vi "Main.vi"() -> ()   [LabVIEW 2013]
uses:
  <vilib>/Instr/_visa.llb/VISA Flush IO Buffer Mask.ctl
  <vilib>/Instr/_visa.llb/VISA Configure Serial Port (Instr).vi
panel:
  out "Roll Array":dbl[](array[numeric])
  out "Pitch Array":dbl[](array[numeric])
  out "Time for Orientation":dbl[](array[numeric])
  out "Time for Temp":dbl[](array[numeric])
  out "Heater Temp":dbl[](array[numeric])
  out "Temp 2":dbl[](array[numeric])
  out "Temp 1":dbl[](array[numeric])
  out "Start time (minutes)":dbl
  out "error out":errorcluster
  in  "error in (no error)":errorcluster
  in  "Tab Control":T1(tab)
  out "Command Recieved":bool
  in  "Reset Relays":bool
  in  "Reset Radio Check":bool
  out "Check Successful!":bool
  in  "Radio Check":bool
  out "Relay 8 Status":bool
  out "Relay 7 Status":bool
  out "Relay 6 Status":bool
  out "Relay 5 Status":bool
  out "Relay 4 Status":bool
  out "Relay 3 Status":bool
  out "Relay 2 Status":bool
  out "Relay 1 Status":bool
  in  "Relay 8":bool
  in  "Relay 7":bool
  in  "Relay 6":bool
  in  "Relay 5":bool
  in  "Relay 4":bool
  in  "Relay 3":bool
  in  "Relay 2":bool
  in  "Relay 1":bool
  out "Manual Heat Control?":bool
  out "Current Time":timestamp format="%<%I:%M:%S %p>T"
  in  "Command":u16(ring) items=["CUTDOWN"=0, "CHANGE_TRANSMIT_RATE"=1, "TURN_HEATER_ON"=2, "TURN_HEATER_OFF"=3, "MANUAL_HEATER_CONTROL"=4, "SWITCH_RELAYS"=100]
  in  "Value":u16
  out "Sensor Specifications Exceeded":bool caption="Warning"
  in  "Stop":bool
  in  "Last Recieved Packet":string
  out "Radio Connection Lost":bool caption="Alarm"
  out "Turbulence":bool caption="Warning"
  in  "Baud Rate":i32=115200
  out "Data Logging OFF":bool caption="Warning"
  in  "Packet Logging File":path
  in  "Log Recieved Packets?":bool=TRUE
  out "Time of Last Recieved Packet":timestamp format="%<%I:%M:%S %p>T"
  out "Heater On?":bool
  out "Yaw":dbl
  out "Roll":dbl
  out "Pitch":dbl
  in  "COM Port":refnum<visa-resource-name>
  in  "Send Command":bool
  in  "Interior Temperature 2":dbl(knob) scale=-60.0..40.0
  out "Relative Humidity":dbl(knob) scale=0.0..100.0
  out "Atmospheric Pressure":dbl(knob) scale=0.0..15.0
  out "Flight Duration":timestamp format="%<%H:%M:%S>T"
  out "Low Interior Temperature":bool caption="Warning"
  out "Critically Low Interior Temperature":bool caption="Alarm"
  in  "Interior Temperature 1":dbl(knob) scale=-60.0..40.0
  in  "Exterior Temperature":dbl(knob) scale=-60.0..40.0
  in  "Heater Temperature":dbl(knob) scale=-60.0..40.0
  out "Yaw":cluster{"X":dbl, "Y":dbl}[](graph)
  out "Atmospheric Pressure":cluster{"X":dbl, "Y":dbl}[](graph)
  out "Exterior Temperature":cluster{"X":dbl, "Y":dbl}[](graph)
  out "Relative Humidity":cluster{"X":dbl, "Y":dbl}[](graph)
  out "Interior Temperature":cluster{dbl[], dbl[]}[](graph)
  out "Pitch/Roll":cluster{dbl[], dbl[]}[](graph)
  in  "Save Packets":bool
  in  "Packet File":path
  out "Packets Recieved":string
  # "Current Instrument Readings"
  # "Relay Status"
  # "Control"
  # "Notes: \n + Relay 1: Tracer 1\n + Relay 2: Unused\n + Relay 3: Unused\n + Relay 4: Heater relay (control blocked)\n\n + Relays 5-8 are not currently wired"
  # "Relays"
  # "See \"Relay Status\"\n panel for relay \nassignments"
  # "Warnings and Alarms"
  # "Communication"
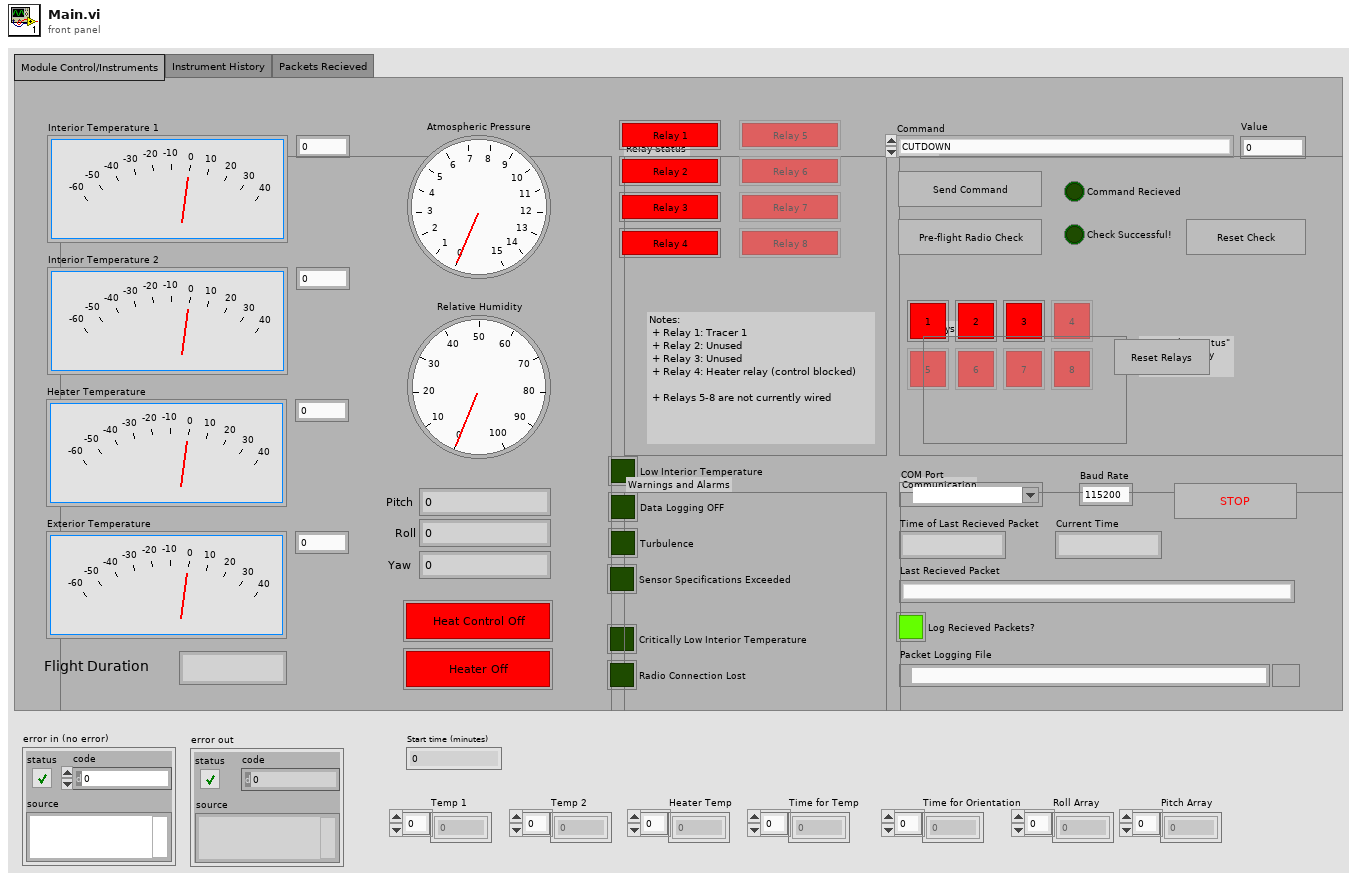
[diagram p1: front panel]
types:
  T1 = enum32{"Module Control/Instruments", "Instrument History", "Packets Recieved"}
  T2 = typedef "VISA Flush IO Buffer Mask.ctl" = u16
  T3 = enum16{"open", "replace", "create", "open or create", "replace or create", "replace or create with confirmation"}
  T4 = cluster{"Digital Interior Temperature":dbl, "Analog Interior Temperature":dbl, "Heater Temperature":dbl, "Exterior Temperature":dbl, "Humidity":dbl, "Pressure":dbl, "Pitch":dbl, "Roll":dbl, "Yaw":dbl, "Heater On?":bool, "Data Logging?":bool, "Manual Heat Control?":bool, "Turbulence":bool, "Relay 1":bool, "Relay 2":bool, "Relay 3":bool, "Relay 4":bool, "Relay 5":bool, "Relay 6":bool, "Relay 7":bool, "Relay 8":bool}
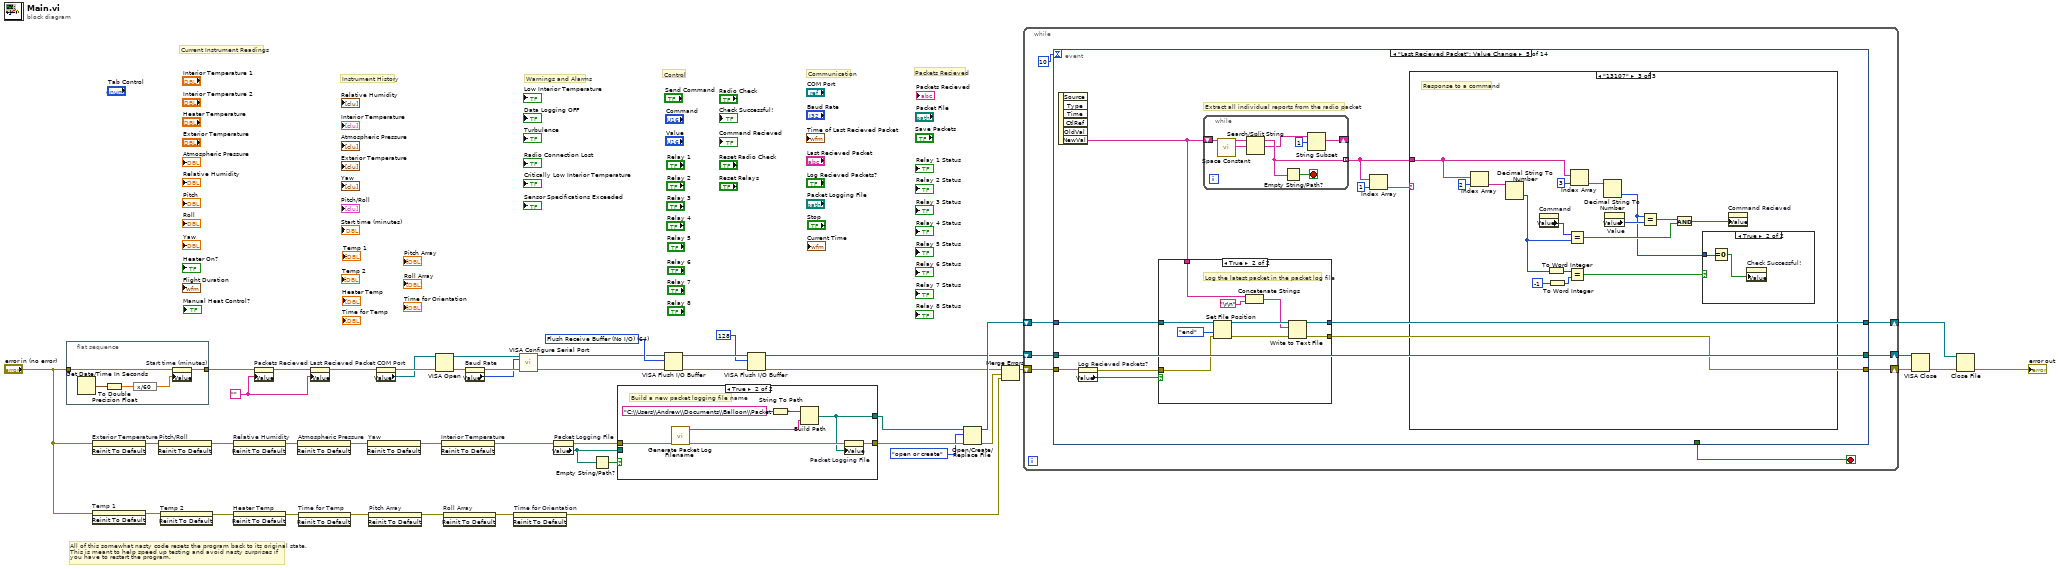
[diagram p0: block diagram]
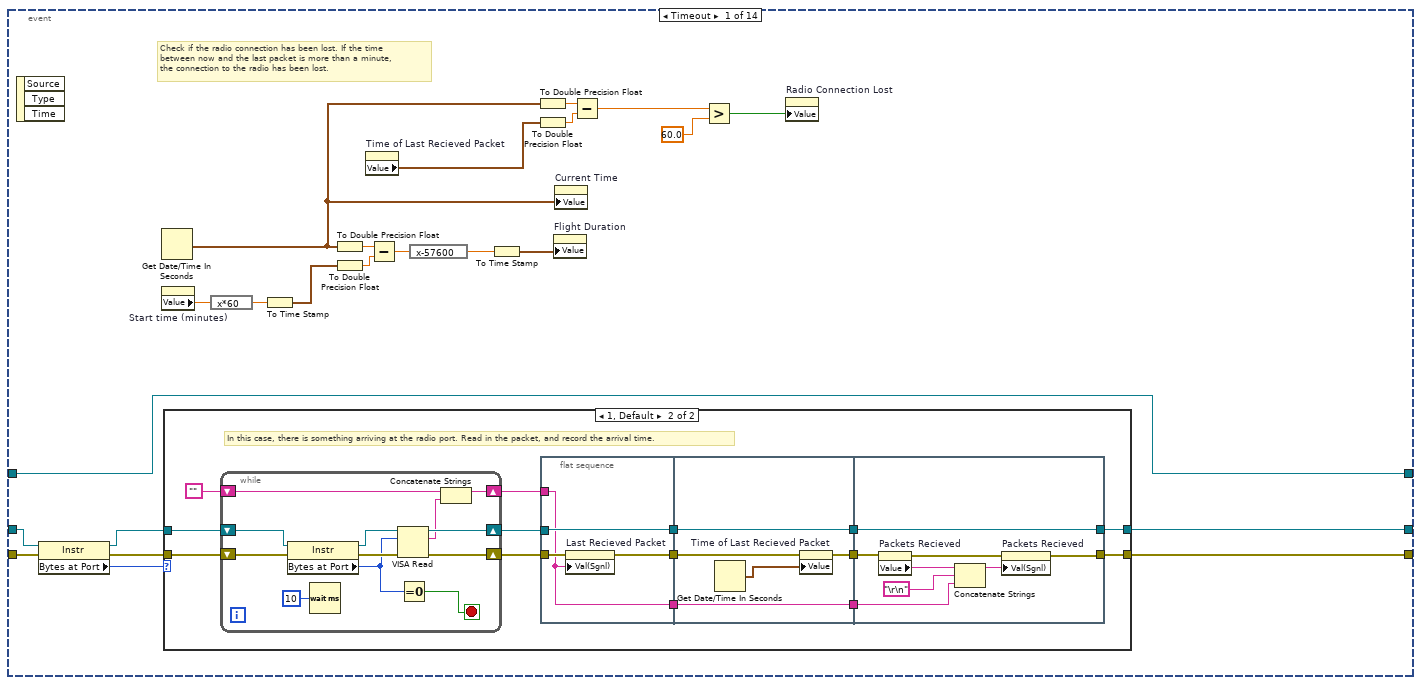
[diagram p3: hidden frame]
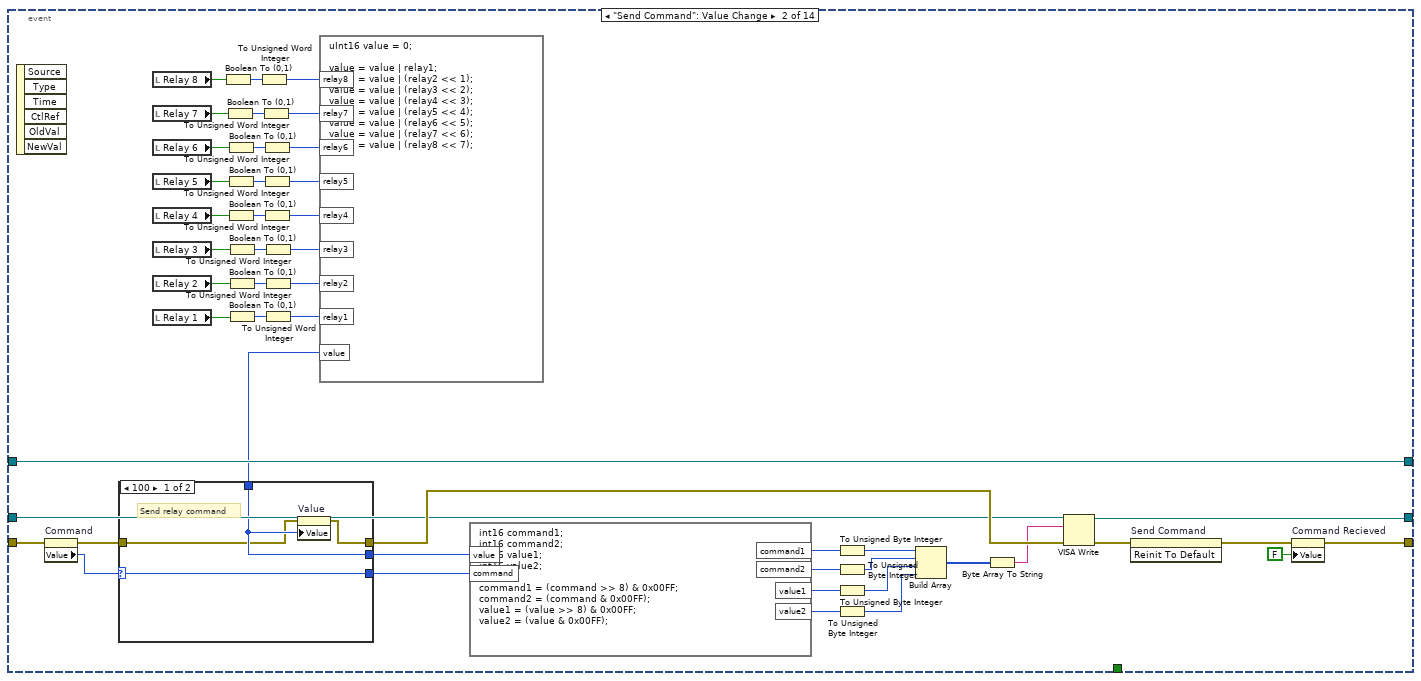
[diagram p5: hidden frame]
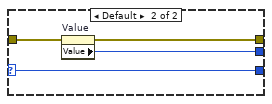
[diagram p6: hidden frame]
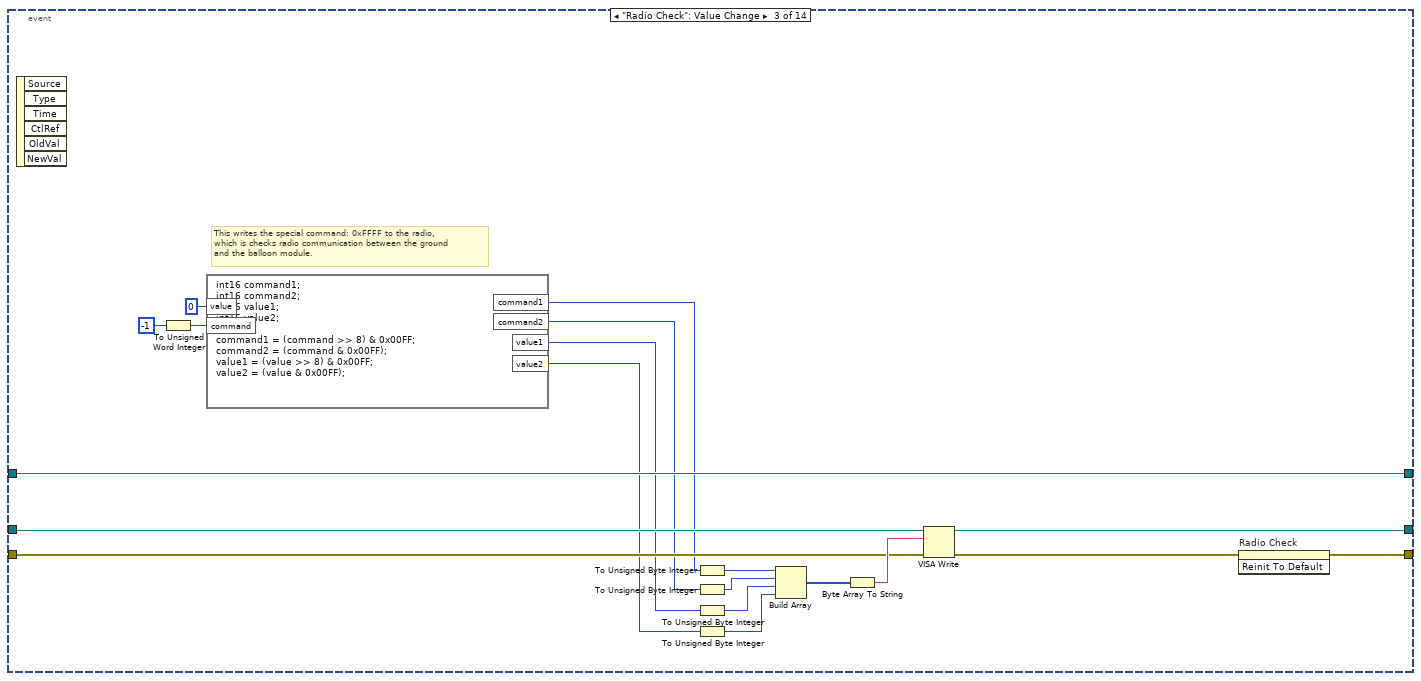
[diagram p7: hidden frame]
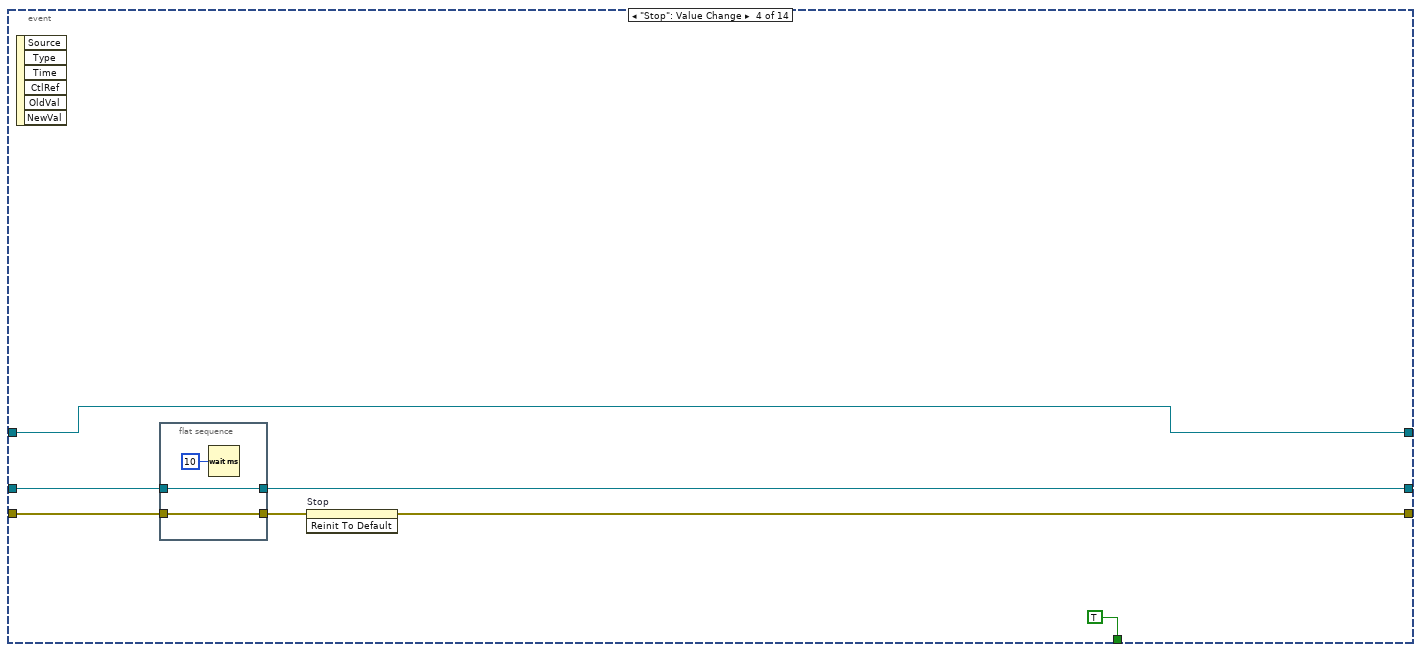
[diagram p8: hidden frame]
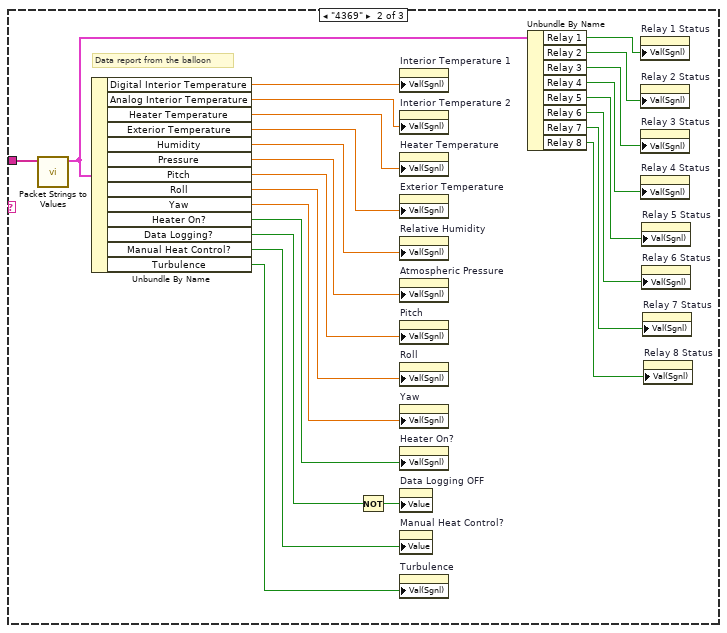
[diagram p10: hidden frame]
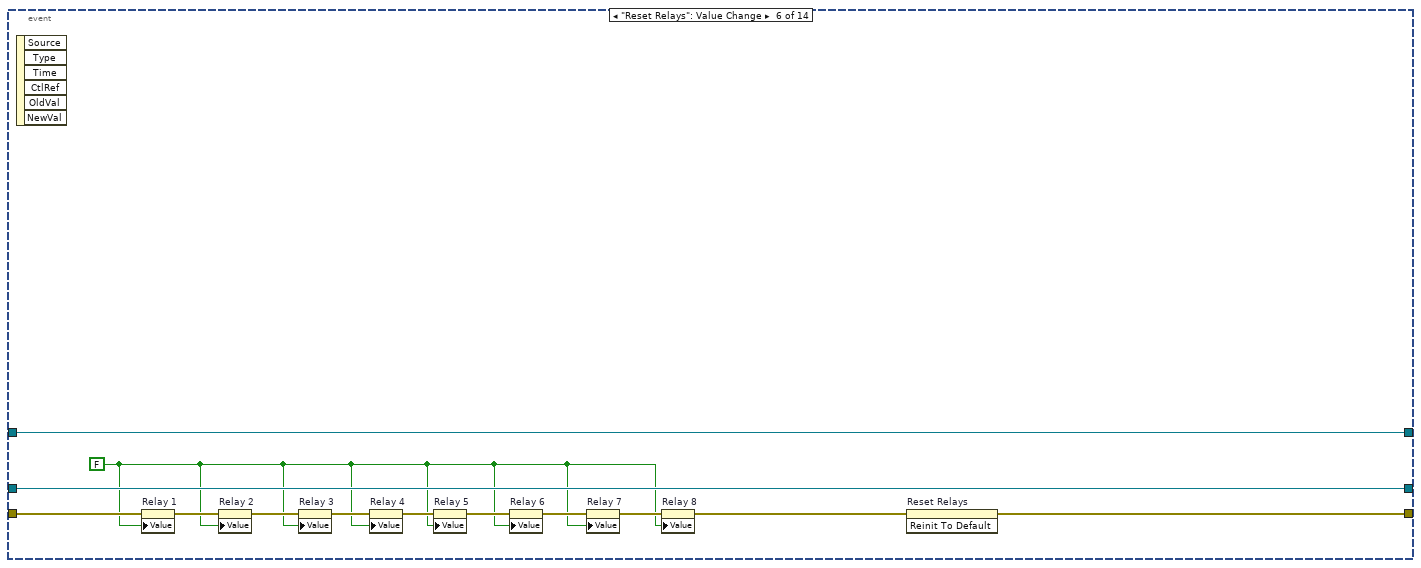
[diagram p13: hidden frame]
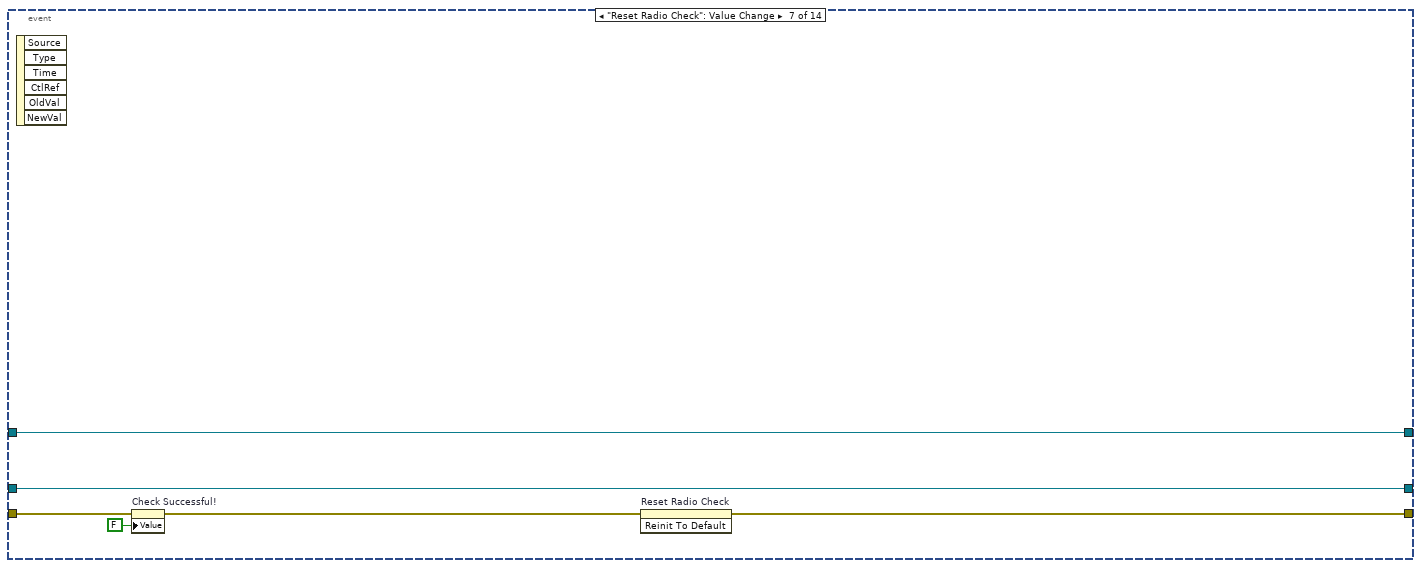
[diagram p14: hidden frame]
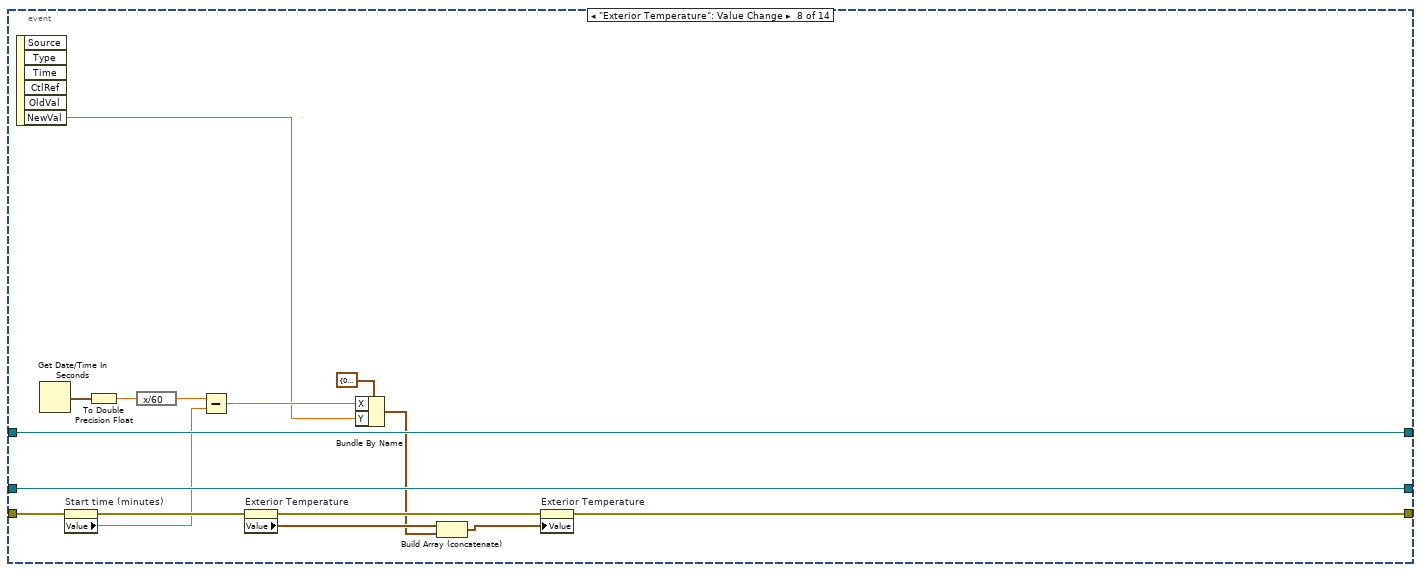
[diagram p15: hidden frame]
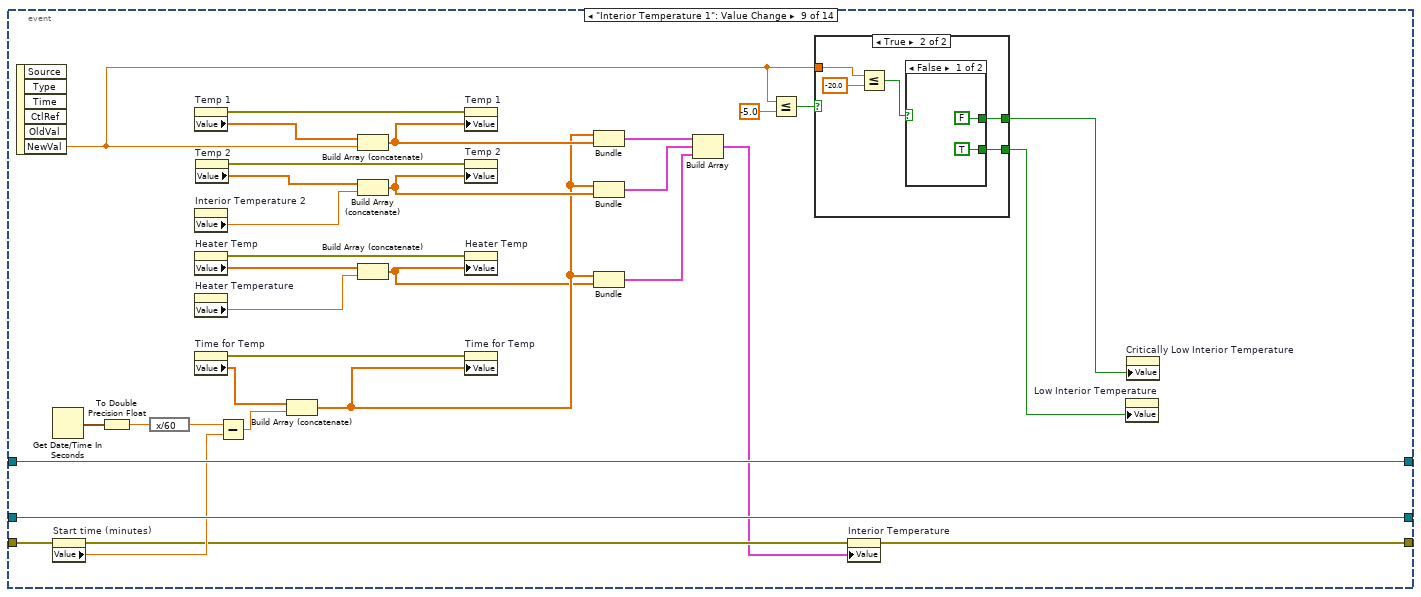
[diagram p16: hidden frame]
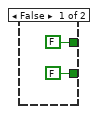
[diagram p17: hidden frame]
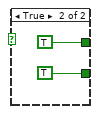
[diagram p18: hidden frame]
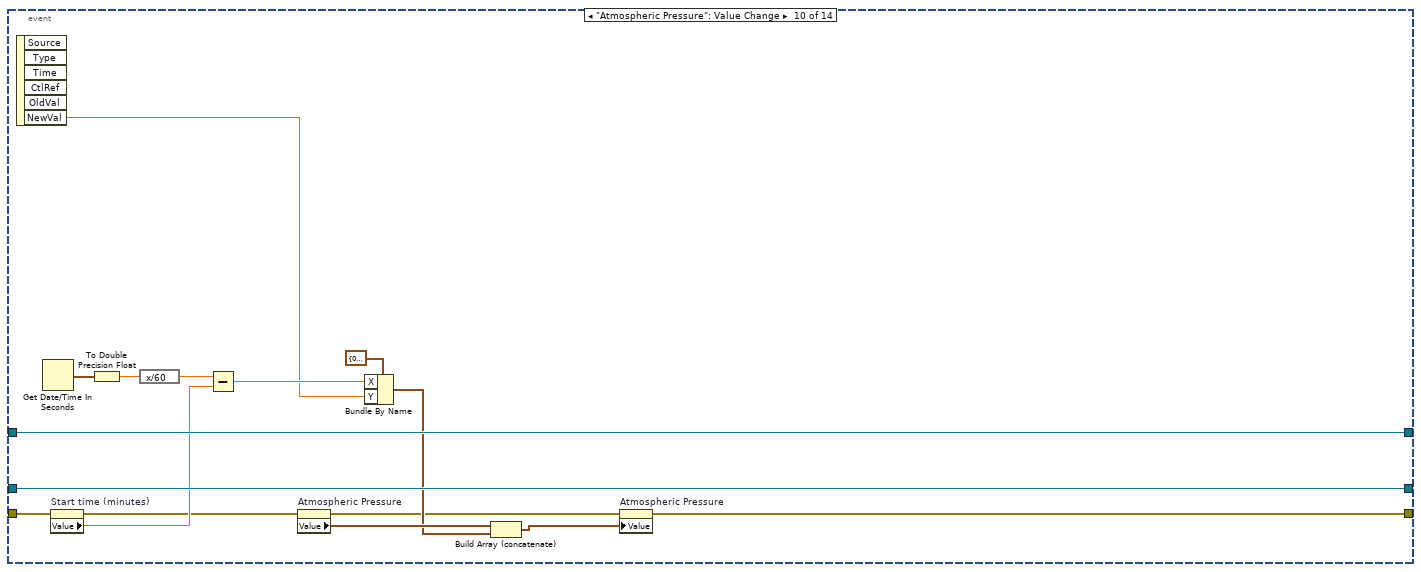
[diagram p19: hidden frame]
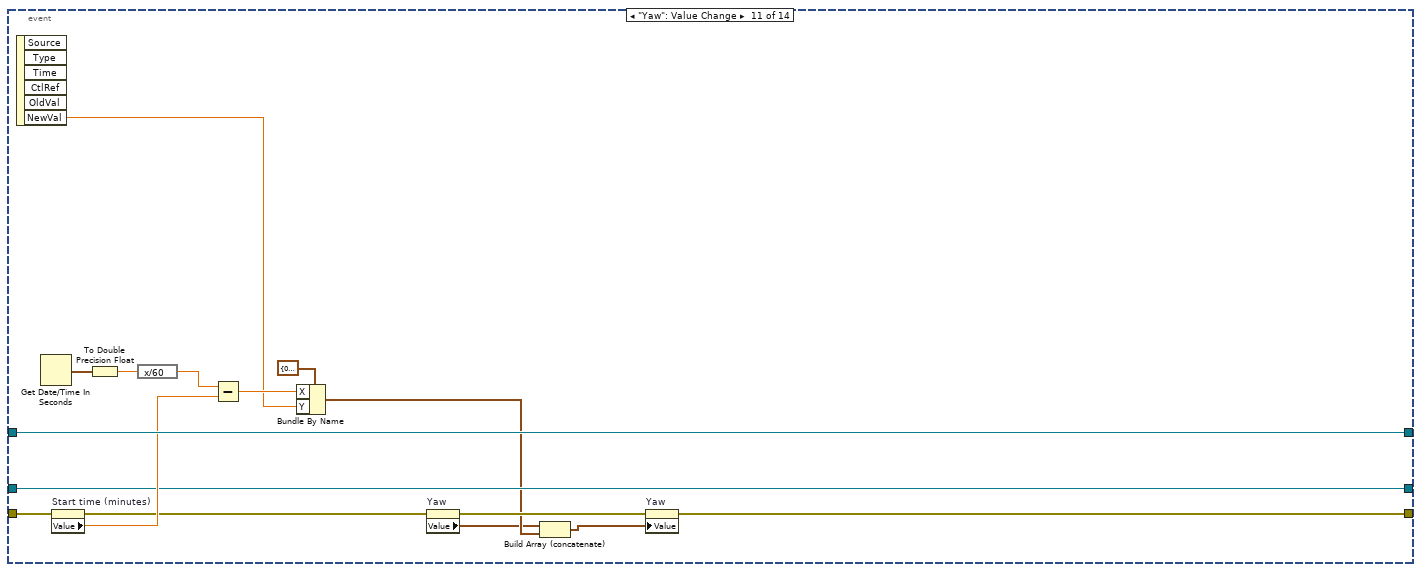
[diagram p20: hidden frame]
diagram:
  w28 = T2 64 items=["Flush Receive Buffer"=16, "Write Transmit Buffer to Device"=32, "Flush Receive Buffer (No I/O)"=64, "Flush Transmit Buffer"=128] ("Mask")
  w17 = ""
  # "All of this somewhat nasty code resets the program back to its original state.\nThis is meant to help speed up testing and avoid nasty surprises if\nyou have to restart the program."
  # "Packets Recieved"
  # "Control"
  # "Communication"
  # "Warnings and Alarms"
  # "Current Instrument Readings"
  # "Instrument History"
  n1 = flat-sequence {
    tunnel: "error in (no error)" -> [w48]
    tunnel: [w49] -> w16
    frame #0 {
      n2 = Get Date/Time In Seconds() -> (seconds since 1Jan1904=w51:timestamp)
      n3 = To Double Precision Float(number=w51) -> (double precision float=w50:dbl)
      n4 = expression code="x/60"(w50) -> (w47:dbl)
      n5 = property on="Start time (minutes)" class="DigNum (strict)"(error in=w48, "Value"=w47) -> (error out=w49:errorcluster)  [unwired: 1 in, 1 out]
    }
  }
  n6 = invoke on="Exterior Temperature" class="XYGraph (strict)" method="Reinit To Default"(error in="error in (no error)") -> (error out=w13:errorcluster)  [unwired: 2 in, 2 out]
  n7 = invoke on="Temp 1" class="Arr (strict)" method="Reinit To Default"(error in="error in (no error)") -> (error out=w9:errorcluster)  [unwired: 2 in, 2 out]
  n8 = invoke on="Pitch/Roll" class="XYGraph (strict)" method="Reinit To Default"(error in=w13) -> (error out=w12:errorcluster)  [unwired: 2 in, 2 out]
  n9 = invoke on="Temp 2" class="Arr (strict)" method="Reinit To Default"(error in=w9) -> (error out=w8:errorcluster)  [unwired: 2 in, 2 out]
  n10 = invoke on="Relative Humidity" class="XYGraph (strict)" method="Reinit To Default"(error in=w12) -> (error out=w15:errorcluster)  [unwired: 2 in, 2 out]
  n11 = invoke on="Heater Temp" class="Arr (strict)" method="Reinit To Default"(error in=w8) -> (error out=w7:errorcluster)  [unwired: 2 in, 2 out]
  n12 = property on="Packets Recieved" class="Str"(error in=w16, "Value"=w17) -> (error out=w19:errorcluster)  [unwired: 1 in, 1 out]
  n13 = invoke on="Atmospheric Pressure" class="XYGraph (strict)" method="Reinit To Default"(error in=w15) -> (error out=w14:errorcluster)  [unwired: 2 in, 2 out]
  n14 = invoke on="Time for Temp" class="Arr (strict)" method="Reinit To Default"(error in=w7) -> (error out=w6:errorcluster)  [unwired: 2 in, 2 out]
  n15 = property on="Last Recieved Packet" class="Str"(error in=w19, "Value"=w17) -> (error out=w18:errorcluster)  [unwired: 1 in, 1 out]
  n16 = invoke on="Yaw" class="XYGraph (strict)" method="Reinit To Default"(error in=w14) -> (error out=w10:errorcluster)  [unwired: 2 in, 2 out]
  n17 = invoke on="Pitch Array" class="Arr (strict)" method="Reinit To Default"(error in=w6) -> (error out=w5:errorcluster)  [unwired: 2 in, 2 out]
  n18 = property on="COM Port" class="VISAName"(error in=w18) -> (error out=w41:errorcluster, "Value"=w40:refnum<visa-resource-name>)  [unwired: 1 in, 1 out]
  n19 = VISA Open(error in (no error)=w41, VISA resource name=w40) -> (VISA resource name=w46:refnum<visa-resource-name>, error out=w44:errorcluster)  [unwired: 3 in]
  n20 = invoke on="Interior Temperature" class="XYGraph (strict)" method="Reinit To Default"(error in=w10) -> (error out=w11:errorcluster)  [unwired: 2 in, 2 out]
  n21 = invoke on="Roll Array" class="Arr (strict)" method="Reinit To Default"(error in=w5) -> (error out=w3:errorcluster)  [unwired: 2 in, 2 out]
  n22 = property on="Baud Rate" class="DigNum (strict)"(error in=w44) -> (error out=w43:errorcluster, "Value"=w42:i32)  [unwired: 1 in, 1 out]
  n23 = invoke on="Time for Orientation" class="Arr (strict)" method="Reinit To Default"(error in=w3) -> (error out=w1:errorcluster)  [unwired: 2 in, 2 out]
  n24 = call-poly "VISA Configure Serial Port"("VISA resource name"=w46, "baud rate (9600)"=w42, "error in (no error)"=w43) -> ("VISA resource name out"=w25:refnum<visa-resource-name>, "error out"=w24:errorcluster)  [unwired: 11 in]
  n25 = property on="Packet Logging File" class="Path"(error in=w11) -> (error out=w37:errorcluster, "Value"=w36:path)  [unwired: 1 in, 1 out]
  n26 = Empty String/Path?(string/path=w36) -> (empty?=w38:bool)
  n27 = case shown="True" w38 {
    tunnel: w37 -> [w53 w60]
    tunnel: [w53 w56] -> w35
    tunnel: [w52 w54] -> w30
    tunnel: w36 -> [w52 _]
    frame False {
    }
    frame True {
      # "Build a new packet logging file name"
      n28 = call "Generate Packet Log Filename.vi"("error in (no error)"=w60) -> ("error out"=w55:errorcluster, "Filename"=w57:string)  [unwired: 9 in]
      n29 = String To Path(string="C:\\Users\\Andrew\\Documents\\Balloon\\Packet Logs") -> (path=w59:path)
      n30 = Build Path(base path=w59, name or relative path=w57) -> (appended path=w54:path)
      n31 = property on="Packet Logging File" class="Path"(error in=w55, "Value"=w54) -> (error out=w56:errorcluster)  [unwired: 1 in, 1 out]
    }
  }
  n32 = VISA Flush I/O Buffer(VISA resource name=w25, mask (16)=w28, error in (no error)=w24) -> (VISA resource name out=w27:refnum<visa-resource-name>, error out=w26:errorcluster)
  n33 = VISA Flush I/O Buffer(VISA resource name=w27, mask (16)=128, error in (no error)=w26) -> (VISA resource name out=w23:refnum<visa-resource-name>, error out=w22:errorcluster)
  n34 = Open/Create/Replace File(file path (use dialog)=w30, error in=w35, operation (0:open)=T3."open or create") -> (refnum out=w29:refnum<file>, error out=w20:errorcluster)  [unwired: 3 in, 1 out]
  n35 = Merge Errors(w22, w20, w1) -> (w21:errorcluster)
  n36 = while {
    shift-right: [w67] -> w45
    shift-left: w21 -> [w68]
    shift-right: [w63] -> w39
    shift-left: w23 -> [w64]
    shift-right: [w61] -> w32
    shift-left: w29 -> [w62]
    stop <- w66 stop-if-true
    n37 = event shown="[4] \"Last Recieved Packet\": Value Change" {
      selector: _ -> [_ _ _ _ _ _ _ _ _ _ _ _ _ _]
      dyn-events: _ -> [_ _ _ _ _ _ _ _ _ _ _ _ _ _]
      timeout: 10 -> [_ _ _ _ _ _ _ _ _ _ _ _ _ _]
      tunnel: w68 -> [w91 w182 w200 w213 w228 w304 w312 w320 w361 w387 w404 w428 w444 w454]
      tunnel: [w87 w138 w211 w216 w229 w294 w309 w325 w338 w375 w389 w414 w435 w446] -> w67
      tunnel: [_ _ _ TRUE _ _ _ _ _ _ _ _ _ _] -> w66
      tunnel: w64 -> [w90 w169 w198 w215 w232 w305 w308 w327 w359 w386 w394 w413 w443 w448]
      tunnel: [w85 w184 w197 w214 w232 w305 w308 w327 w359 w386 w394 w413 w443 w447] -> w63
      tunnel: w62 -> [w84 w183 w210 w212 w231 w306 w307 w328 w360 w388 w403 w427 w438 w450]
      tunnel: [w84 w183 w210 w212 w230 w306 w307 w328 w360 w388 w403 w427 w438 w449] -> w61
      event Timeout {
        # "Check if the radio connection has been lost. If the time \nbetween now and the last packet is more than a minute,\nthe connection to the radio has been lost."
        n38 = event-data() -> ()  [unwired: 1 in, 3 out]
        n39 = property class="Instr"(reference=w90, error in=w91) -> (reference out=w86:refnum<visa-resource-name>, error out=w88:errorcluster, "Bytes at Port"=w89:u32)
        n40 = Get Date/Time In Seconds() -> (seconds since 1Jan1904=w73:timestamp)
        n41 = property on="Start time (minutes)" class="DigNum (strict)"() -> ("Value"=w83:dbl)  [unwired: 2 in, 2 out]
        n42 = case shown="1, Default" w89 {
          tunnel: w88 -> [w92 w98]
          tunnel: [w92 w104] -> w87
          tunnel: w86 -> [w93 w99]
          tunnel: [w93 w105] -> w85
          frame 0 {
            # "No packets are waiting to be read in the radio port."
          }
          frame 1, Default {
            # "In this case, there is something arriving at the radio port. Read in the packet, and record the arrival time."
            n43 = while {
              shift-right: [w115] -> w97
              shift-left: w99 -> [w117]
              shift-right: [w114] -> w96
              shift-left: w98 -> [w119]
              shift-right: [w110] -> w94
              shift-left: "" -> [w111]
              stop <- w112 stop-if-true
              n44 = property class="Instr"(reference=w117, error in=w119) -> (reference out=w116:refnum<visa-resource-name>, error out=w118:errorcluster, "Bytes at Port"=w113:u32)
              n45 = Wait (ms)(milliseconds to wait=u32 10) -> ()  [unwired: 1 out]
              n46 = VISA Read(VISA resource name=w116, byte count=w113, error in (no error)=w118) -> (VISA resource name out=w115:refnum<visa-resource-name>, read buffer=w109:string, error out=w114:errorcluster)  [unwired: 1 out]
              n47 = Equal To 0?(x=w113) -> (x = 0?=w112:bool)
              n48 = Concatenate Strings(w111, w109) -> (w110:string)
            }
            n49 = flat-sequence {
              tunnel: w96 -> [w121]
              tunnel: w97 -> [w122]
              tunnel: [w122] -> w107
              tunnel: [w123] -> w106
              tunnel: [w120] -> w100
              tunnel: w94 -> [w120]
              tunnel: w107 -> [w127]
              tunnel: w106 -> [w128]
              tunnel: [w127] -> w103
              tunnel: [w126] -> w102
              tunnel: [w124] -> w101
              tunnel: w100 -> [w124]
              tunnel: [w130] -> w104
              tunnel: [w136] -> w105
              tunnel: w103 -> [w136]
              tunnel: w102 -> [w131]
              tunnel: w101 -> [w129]
              frame #0 {
                n50 = property on="Last Recieved Packet" class="Str"(error in=w121, "Val(Sgnl)"=w120) -> (error out=w123:errorcluster)  [unwired: 1 in, 1 out]
              }
              frame #1 {
                n51 = Get Date/Time In Seconds() -> (seconds since 1Jan1904=w125:timestamp)
                n52 = property on="Time of Last Recieved Packet" class="AbsTime (strict)"(error in=w128, "Value"=w125) -> (error out=w126:errorcluster)  [unwired: 1 in, 1 out]
              }
              frame #2 {
                n53 = property on="Packets Recieved" class="Str"(error in=w131) -> (error out=w134:errorcluster, "Value"=w132:string)  [unwired: 1 in, 1 out]
                n54 = Concatenate Strings(w132, "\r\n", w129) -> (w135:string)
                n55 = property on="Packets Recieved" class="Str"(error in=w134, "Val(Sgnl)"=w135) -> (error out=w130:errorcluster)  [unwired: 1 in, 1 out]
              }
            }
          }
        }
        n56 = expression code="x*60"(w83) -> (w82:dbl)
        n57 = To Time Stamp(1:w82) -> (0:w79:timestamp)
        n58 = To Double Precision Float(number=w73) -> (double precision float=w80:dbl)
        n59 = To Double Precision Float(number=w79) -> (double precision float=w78:dbl)
        n60 = property on="Time of Last Recieved Packet" class="AbsTime (strict)"() -> ("Value"=w72:timestamp)  [unwired: 2 in, 2 out]
        n61 = Subtract(x=w80, y=w78) -> (x-y=w77:dbl)
        n62 = expression code="x-57600"(w77) -> (w76:dbl)
        n63 = To Time Stamp(1:w76) -> (0:w81:timestamp)
        n64 = To Double Precision Float(number=w73) -> (double precision float=w75:dbl)
        n65 = To Double Precision Float(number=w72) -> (double precision float=w74:dbl)
        n66 = property on="Flight Duration" class="AbsTime (strict)"("Value"=w81) -> ()  [unwired: 2 in, 2 out]
        n67 = property on="Current Time" class="AbsTime (strict)"("Value"=w73) -> ()  [unwired: 2 in, 2 out]
        n68 = Subtract(x=w75, y=w74) -> (x-y=w69:dbl)
        n69 = Greater?(x=w69, y=60.0) -> (0:w70:bool)
        n70 = property on="Radio Connection Lost" class="Bool (strict)"("Value"=w70) -> ()  [unwired: 2 in, 2 out]
      }
      event "Send Command": Value Change {
        n71 = event-data() -> ()  [unwired: 1 in, 6 out]
        n72 = property on="Command" class="Ring (strict)"(error in=w182) -> (error out=w181:errorcluster, "Value"=w166:u16)  [unwired: 1 in, 1 out]
        n73 = local read "Relay 8"() -> (w163:bool)
        n74 = local read "Relay 7"() -> (w161:bool)
        n75 = local read "Relay 6"() -> (w159:bool)
        n76 = local read "Relay 5"() -> (w157:bool)
        n77 = local read "Relay 4"() -> (w155:bool)
        n78 = local read "Relay 3"() -> (w153:bool)
        n79 = local read "Relay 2"() -> (w151:bool)
        n80 = local read "Relay 1"() -> (w149:bool)
        n81 = Boolean To (0,1)(Boolean=w163) -> (0, 1=w164:i16)
        n82 = Boolean To (0,1)(Boolean=w161) -> (0, 1=w162:i16)
        n83 = Boolean To (0,1)(Boolean=w159) -> (0, 1=w160:i16)
        n84 = Boolean To (0,1)(Boolean=w157) -> (0, 1=w158:i16)
        n85 = Boolean To (0,1)(Boolean=w155) -> (0, 1=w156:i16)
        n86 = Boolean To (0,1)(Boolean=w153) -> (0, 1=w154:i16)
        n87 = Boolean To (0,1)(Boolean=w151) -> (0, 1=w152:i16)
        n88 = Boolean To (0,1)(Boolean=w149) -> (0, 1=w150:i16)
        n89 = To Unsigned Word Integer(number=w164) -> (unsigned 16bit integer=w141:u16)
        n90 = To Unsigned Word Integer(number=w162) -> (unsigned 16bit integer=w142:u16)
        n91 = To Unsigned Word Integer(number=w160) -> (unsigned 16bit integer=w143:u16)
        n92 = To Unsigned Word Integer(number=w158) -> (unsigned 16bit integer=w144:u16)
        n93 = To Unsigned Word Integer(number=w156) -> (unsigned 16bit integer=w145:u16)
        n94 = To Unsigned Word Integer(number=w154) -> (unsigned 16bit integer=w146:u16)
        n95 = To Unsigned Word Integer(number=w152) -> (unsigned 16bit integer=w148:u16)
        n96 = To Unsigned Word Integer(number=w150) -> (unsigned 16bit integer=w147:u16)
        n97 = formula code="uInt16 value = 0;\n\nvalue = value | relay1;\nvalue = value | (relay2 << 1);\nvalue = value | (relay3 << 2);\nvalue = value | (relay4 << 3);\nvalue = value | (relay5 << 4);\nvalue = value | (relay6 << 5);\nvalue = value | (relay7 << 6);\nvalue = value | (relay8 << 7);"("relay1"=w147, "relay2"=w148, "relay3"=w146, "relay4"=w145, "relay5"=w144, "relay6"=w143, "relay7"=w142, "relay8"=w141) -> ("value"=w140:u16)
        n98 = case shown="100" w166 {
          selector: w166 -> [w188 w189]
          tunnel: w181 -> [w185 w192]
          tunnel: [w186 w191] -> w180
          tunnel: [w187 w190] -> w171
          tunnel: [w188 w189] -> w165
          tunnel: w140 -> [w186 _]
          frame 100 {
            # "Send relay command"
            n99 = property on="Value" class="DigNum (strict)"(error in=w185, "Value"=w186) -> (error out=w187:errorcluster)  [unwired: 1 in, 1 out]
          }
          frame Default {
            n100 = property on="Value" class="DigNum (strict)"(error in=w192) -> (error out=w190:errorcluster, "Value"=w191:u16)  [unwired: 1 in, 1 out]
          }
        }
        n101 = formula code="int16 command1;\nint16 command2;\nint16 value1;\nint16 value2;\n\ncommand1 = (command >> 8) & 0x00FF;\ncommand2 = (command & 0x00FF);\nvalue1 = (value >> 8) & 0x00FF;\nvalue2 = (value & 0x00FF);"("command"=w165, "value"=w180) -> ("command1"=w178:i16, "command2"=w177:i16, "value1"=w176:i16, "value2"=w175:i16)
        n102 = To Unsigned Byte Integer(number=w178) -> (unsigned 8bit integer=w179:u8)
        n103 = To Unsigned Byte Integer(number=w177) -> (unsigned 8bit integer=w174:u8)
        n104 = To Unsigned Byte Integer(number=w176) -> (unsigned 8bit integer=w173:u8)
        n105 = To Unsigned Byte Integer(number=w175) -> (unsigned 8bit integer=w172:u8)
        n106 = Build Array(w179, w174, w173, w172) -> (w167:u8[])
        n107 = Byte Array To String(unsigned byte array=w167) -> (string=w170:string)
        n108 = VISA Write(VISA resource name=w169, write buffer=w170, error in (no error)=w171) -> (VISA resource name out=w184:refnum<visa-resource-name>, error out=w168:errorcluster)  [unwired: 1 out]
        n109 = invoke on="Send Command" class="Bool" method="Reinit To Default"(error in=w168) -> (error out=w139:errorcluster)  [unwired: 2 in, 2 out]
        n110 = property on="Command Recieved" class="Bool (strict)"(error in=w139, "Value"=FALSE ("Command Recieved")) -> (error out=w138:errorcluster)  [unwired: 1 in, 1 out]
      }
      event "Radio Check": Value Change {
        # "This writes the special command: 0xFFFF to the radio,\nwhich is checks radio communication between the ground\nand the balloon module."
        n111 = event-data() -> ()  [unwired: 1 in, 6 out]
        n112 = To Unsigned Word Integer(number=-1) -> (unsigned 16bit integer=w208:u16)
        n113 = formula code="int16 command1;\nint16 command2;\nint16 value1;\nint16 value2;\n\ncommand1 = (command >> 8) & 0x00FF;\ncommand2 = (command & 0x00FF);\nvalue1 = (value >> 8) & 0x00FF;\nvalue2 = (value & 0x00FF);"("command"=w208, "value"=u16 0 ("input variable")) -> ("command1"=w196:i16, "command2"=w195:i16, "value1"=w194:i16, "value2"=w193:i16)
        n114 = To Unsigned Byte Integer(number=w196) -> (unsigned 8bit integer=w201:u8)
        n115 = To Unsigned Byte Integer(number=w195) -> (unsigned 8bit integer=w202:u8)
        n116 = To Unsigned Byte Integer(number=w194) -> (unsigned 8bit integer=w203:u8)
        n117 = To Unsigned Byte Integer(number=w193) -> (unsigned 8bit integer=w204:u8)
        n118 = Build Array(w201, w202, w203, w204) -> (w206:u8[])
        n119 = Byte Array To String(unsigned byte array=w206) -> (string=w205:string)
        n120 = VISA Write(VISA resource name=w198, write buffer=w205, error in (no error)=w200) -> (VISA resource name out=w197:refnum<visa-resource-name>, error out=w199:errorcluster)  [unwired: 1 out]
        n121 = invoke on="Radio Check" class="Bool" method="Reinit To Default"(error in=w199) -> (error out=w211:errorcluster)  [unwired: 2 in, 2 out]
      }
      event "Stop": Value Change {
        n122 = event-data() -> ()  [unwired: 1 in, 6 out]
        n123 = flat-sequence {
          tunnel: w213 -> [w220]
          tunnel: [w220] -> w217
          tunnel: w215 -> [w219]
          tunnel: [w219] -> w214
          frame #0 {
            n124 = Wait (ms)(milliseconds to wait=u32 10) -> ()  [unwired: 1 out]
          }
        }
        n125 = invoke on="Stop" class="Bool" method="Reinit To Default"(error in=w217) -> (error out=w216:errorcluster)  [unwired: 2 in, 2 out]
      }
      event "Last Recieved Packet": Value Change {
        # "Extract all individual reports from the radio packet"
        n126 = event-data() -> ("NewVal"=w225:string)  [unwired: 1 in, 5 out]
        n127 = property on="Log Recieved Packets?" class="Bool (strict)"(error in=w228) -> (error out=w227:errorcluster, "Value"=w226:bool)  [unwired: 1 in, 1 out]
        n128 = case shown="True" w226 {
          tunnel: w231 -> [w283 w290]
          tunnel: [w283 w289] -> w230
          tunnel: [w282 w288] -> w229
          tunnel: w227 -> [w282 w287]
          tunnel: w225 -> [_ w286]
          frame False {
            # "We don't want to log the packets, so do nothing"
          }
          frame True {
            # "Log the latest packet in the packet log file"
            n129 = Set File Position(refnum=w290, from (0:start)=enum16{"start", "end", "current"}."end", error in=w287) -> (refnum out=w291:refnum<file>, error out=w292:errorcluster)  [unwired: 1 in]
            n130 = Concatenate Strings(w286, "\r\n") -> (w284:string)
            n131 = Write to Text File(file (use dialog)=w291, text=w284, error in=w292) -> (refnum out=w289:refnum<file>, error out=w288:errorcluster)  [unwired: 1 in, 1 out]
          }
        }
        n132 = while {
          shift-right: [w275] -> _
          shift-left: w225 -> [w280]
          tunnel: [w278] -> w222 mode=indexing
          stop <- w281 stop-if-true
          n133 = call <vilib>:"Space Constant.vi"() -> ("String"=w279:string)
          n134 = Search/Split String(string=w280, search string/char (-)=w279) -> (substring before match=w278:string, match + rest of string=w277:string)  [unwired: 1 in, 1 out]
          n135 = Empty String/Path?(string/path=w278) -> (empty?=w281:bool)
          n136 = String Subset(string=w277, offset (0)=1) -> (substring=w275:string)  [unwired: 1 in]
        }
        n137 = Index Array(array=w222, index=1) -> (element=w223:string)
        n138 = case shown="\"13107\"" w223 {
          tunnel: w222 -> [_ w256 w271]
          frame Default {
            # "Some unrecognized value... do nothing"
          }
          frame "4369" {
            # "Data report from the balloon"
            n139 = call "Packet Strings to Values.vi"("Pakcet Values"=w256) -> ("Data Report"=w241:T4)  [unwired: 10 in]
            n140 = Unbundle By Name(w241) -> ("Digital Interior Temperature"=w255:dbl, "Analog Interior Temperature"=w254:dbl, "Heater Temperature"=w253:dbl, "Exterior Temperature"=w252:dbl, "Humidity"=w251:dbl, "Pressure"=w250:dbl, "Pitch"=w249:dbl, "Roll"=w248:dbl, "Yaw"=w247:dbl, "Heater On?"=w246:bool, "Data Logging?"=w243:bool, "Manual Heat Control?"=w245:bool, "Turbulence"=w242:bool)
            n141 = Not(x=w243) -> (.not. x?=w244:bool)
            n142 = property on="Interior Temperature 1" class="Knob (strict)"("Val(Sgnl)"=w255) -> ()  [unwired: 2 in, 2 out]
            n143 = property on="Interior Temperature 2" class="Knob (strict)"("Val(Sgnl)"=w254) -> ()  [unwired: 2 in, 2 out]
            n144 = property on="Heater Temperature" class="Knob (strict)"("Val(Sgnl)"=w253) -> ()  [unwired: 2 in, 2 out]
            n145 = property on="Exterior Temperature" class="Knob (strict)"("Val(Sgnl)"=w252) -> ()  [unwired: 2 in, 2 out]
            n146 = property on="Relative Humidity" class="Knob (strict)"("Val(Sgnl)"=w251) -> ()  [unwired: 2 in, 2 out]
            n147 = property on="Atmospheric Pressure" class="Knob (strict)"("Val(Sgnl)"=w250) -> ()  [unwired: 2 in, 2 out]
            n148 = property on="Pitch" class="DigNum (strict)"("Val(Sgnl)"=w249) -> ()  [unwired: 2 in, 2 out]
            n149 = property on="Roll" class="DigNum (strict)"("Val(Sgnl)"=w248) -> ()  [unwired: 2 in, 2 out]
            n150 = property on="Yaw" class="DigNum (strict)"("Val(Sgnl)"=w247) -> ()  [unwired: 2 in, 2 out]
            n151 = property on="Heater On?" class="Bool (strict)"("Val(Sgnl)"=w246) -> ()  [unwired: 2 in, 2 out]
            n152 = property on="Data Logging OFF" class="Bool (strict)"("Value"=w244) -> ()  [unwired: 2 in, 2 out]
            n153 = property on="Manual Heat Control?" class="Bool (strict)"("Value"=w245) -> ()  [unwired: 2 in, 2 out]
            n154 = property on="Turbulence" class="Bool (strict)"("Val(Sgnl)"=w242) -> ()  [unwired: 2 in, 2 out]
            n155 = Unbundle By Name(w241) -> ("Relay 1"=w240:bool, "Relay 2"=w239:bool, "Relay 3"=w238:bool, "Relay 4"=w237:bool, "Relay 5"=w236:bool, "Relay 6"=w235:bool, "Relay 7"=w233:bool, "Relay 8"=w234:bool)
            n156 = property on="Relay 1 Status" class="Bool (strict)"("Val(Sgnl)"=w240) -> ()  [unwired: 2 in, 2 out]
            n157 = property on="Relay 2 Status" class="Bool (strict)"("Val(Sgnl)"=w239) -> ()  [unwired: 2 in, 2 out]
            n158 = property on="Relay 3 Status" class="Bool (strict)"("Val(Sgnl)"=w238) -> ()  [unwired: 2 in, 2 out]
            n159 = property on="Relay 4 Status" class="Bool (strict)"("Val(Sgnl)"=w237) -> ()  [unwired: 2 in, 2 out]
            n160 = property on="Relay 5 Status" class="Bool (strict)"("Val(Sgnl)"=w236) -> ()  [unwired: 2 in, 2 out]
            n161 = property on="Relay 6 Status" class="Bool (strict)"("Val(Sgnl)"=w235) -> ()  [unwired: 2 in, 2 out]
            n162 = property on="Relay 7 Status" class="Bool (strict)"("Val(Sgnl)"=w233) -> ()  [unwired: 2 in, 2 out]
            n163 = property on="Relay 8 Status" class="Bool (strict)"("Val(Sgnl)"=w234) -> ()  [unwired: 2 in, 2 out]
          }
          frame "13107" {
            # "Response to a command"
            n164 = Index Array(array=w271, index=2) -> (element=w269:string)
            n165 = Decimal String To Number(string=w269) -> (number=w265:i32)  [unwired: 2 in, 1 out]
            n166 = property on="Command" class="Ring (strict)"() -> ("Value"=w266:u16)  [unwired: 2 in, 2 out]
            n167 = To Word Integer(number=w265) -> (16bit integer=w267:i16)
            n168 = To Word Integer(number=-1) -> (16bit integer=w258:i16)
            n169 = Equal?(x=w266, y=w265) -> (x = y?=w262:bool)
            n170 = Equal?(x=w267, y=w258) -> (x = y?=w261:bool)
            n171 = Index Array(array=w271, index=3) -> (element=w268:string)
            n172 = Decimal String To Number(string=w268) -> (number=w257:i32)  [unwired: 2 in, 1 out]
            n173 = property on="Value" class="DigNum (strict)"() -> ("Value"=w264:u16)  [unwired: 2 in, 2 out]
            n174 = Equal?(x=w257, y=w264) -> (x = y?=w263:bool)
            n175 = And(x=w263, y=w262) -> (x .and. y?=w260:bool)
            n176 = case shown="True" w261 {
              tunnel: w257 -> [_ w274]
              frame False {
              }
              frame True {
                n177 = Equal To 0?(x=w274) -> (x = 0?=w273:bool)
                n178 = property on="Check Successful!" class="Bool (strict)"("Value"=w273) -> ()  [unwired: 2 in, 2 out]
              }
            }
            n179 = property on="Command Recieved" class="Bool (strict)"("Value"=w260) -> ()  [unwired: 2 in, 2 out]
          }
        }
      }
      event "Reset Relays": Value Change {
        w296 = FALSE
        n180 = event-data() -> ()  [unwired: 1 in, 6 out]
        n181 = property on="Relay 1" class="Bool (strict)"(error in=w304, "Value"=w296) -> (error out=w303:errorcluster)  [unwired: 1 in, 1 out]
        n182 = property on="Relay 2" class="Bool (strict)"(error in=w303, "Value"=w296) -> (error out=w302:errorcluster)  [unwired: 1 in, 1 out]
        n183 = property on="Relay 3" class="Bool (strict)"(error in=w302, "Value"=w296) -> (error out=w301:errorcluster)  [unwired: 1 in, 1 out]
        n184 = property on="Relay 4" class="Bool (strict)"(error in=w301, "Value"=w296) -> (error out=w300:errorcluster)  [unwired: 1 in, 1 out]
        n185 = property on="Relay 5" class="Bool (strict)"(error in=w300, "Value"=w296) -> (error out=w299:errorcluster)  [unwired: 1 in, 1 out]
        n186 = property on="Relay 6" class="Bool (strict)"(error in=w299, "Value"=w296) -> (error out=w298:errorcluster)  [unwired: 1 in, 1 out]
        n187 = property on="Relay 7" class="Bool (strict)"(error in=w298, "Value"=w296) -> (error out=w297:errorcluster)  [unwired: 1 in, 1 out]
        n188 = property on="Relay 8" class="Bool (strict)"(error in=w297, "Value"=w296) -> (error out=w295:errorcluster)  [unwired: 1 in, 1 out]
        n189 = invoke on="Reset Relays" class="Bool" method="Reinit To Default"(error in=w295) -> (error out=w294:errorcluster)  [unwired: 2 in, 2 out]
      }
      event "Reset Radio Check": Value Change {
        n190 = event-data() -> ()  [unwired: 1 in, 6 out]
        n191 = property on="Check Successful!" class="Bool (strict)"(error in=w312, "Value"=FALSE ("Check Successful!")) -> (error out=w310:errorcluster)  [unwired: 1 in, 1 out]
        n192 = invoke on="Reset Radio Check" class="Bool" method="Reinit To Default"(error in=w310) -> (error out=w309:errorcluster)  [unwired: 2 in, 2 out]
      }
      event "Exterior Temperature": Value Change {
        n193 = event-data() -> ("NewVal"=w315:dbl)  [unwired: 1 in, 5 out]
        n194 = Get Date/Time In Seconds() -> (seconds since 1Jan1904=w321:timestamp)
        n195 = property on="Start time (minutes)" class="DigNum (strict)"(error in=w320) -> (error out=w319:errorcluster, "Value"=w317:dbl)  [unwired: 1 in, 1 out]
        n196 = To Double Precision Float(number=w321) -> (double precision float=w322:dbl)
        n197 = expression code="x/60"(w322) -> (w318:dbl)
        n198 = Subtract(x=w318, y=w317) -> (x-y=w316:dbl)
        n199 = property on="Exterior Temperature" class="XYGraph (strict)"(error in=w319) -> (error out=w326:errorcluster, "Value"=w324:cluster{"X":dbl, "Y":dbl}[])  [unwired: 1 in, 1 out]
        n200 = Bundle By Name(cluster=cluster{"X":dbl, "Y":dbl} {"X"=0.0, "Y"=0.0} ("element"), "X"=w316, "Y"=w315) -> (w314:cluster{"X":dbl, "Y":dbl})
        n201 = Build Array (concatenate)(w324, w314) -> (w313:cluster{"X":dbl, "Y":dbl}[])
        n202 = property on="Exterior Temperature" class="XYGraph (strict)"(error in=w326, "Value"=w313) -> (error out=w325:errorcluster)  [unwired: 1 in, 1 out]
      }
      event "Interior Temperature 1": Value Change {
        n203 = event-data() -> ("NewVal"=w331:dbl)  [unwired: 1 in, 5 out]
        n204 = Get Date/Time In Seconds() -> (seconds since 1Jan1904=w357:timestamp)
        n205 = property on="Start time (minutes)" class="DigNum (strict)"(error in=w361) -> (error out=w340:errorcluster, "Value"=w355:dbl)  [unwired: 1 in, 1 out]
        n206 = To Double Precision Float(number=w357) -> (double precision float=w356:dbl)
        n207 = expression code="x/60"(w356) -> (w358:dbl)
        n208 = property on="Temp 1" class="Arr (strict)"() -> (error out=w346:errorcluster, "Value"=w349:dbl[])  [unwired: 2 in, 1 out]
        n209 = property on="Interior Temperature 2" class="Knob (strict)"() -> ("Value"=w351:dbl)  [unwired: 2 in, 2 out]
        n210 = property on="Heater Temp" class="Arr (strict)"() -> (error out=w344:errorcluster, "Value"=w347:dbl[])  [unwired: 2 in, 1 out]
        n211 = property on="Heater Temperature" class="Knob (strict)"() -> ("Value"=w350:dbl)  [unwired: 2 in, 2 out]
        n212 = property on="Time for Temp" class="Arr (strict)"() -> (error out=w352:errorcluster, "Value"=w353:dbl[])  [unwired: 2 in, 1 out]
        n213 = property on="Temp 2" class="Arr (strict)"() -> (error out=w345:errorcluster, "Value"=w348:dbl[])  [unwired: 2 in, 1 out]
        n214 = Subtract(x=w358, y=w355) -> (x-y=w354:dbl)
        n215 = Build Array (concatenate)(w353, w354) -> (w335:dbl[])
        n216 = Build Array (concatenate)(w349, w331) -> (w337:dbl[])
        n217 = Build Array (concatenate)(w348, w351) -> (w336:dbl[])
        n218 = Build Array (concatenate)(w347, w350) -> (w334:dbl[])
        n219 = property on="Temp 1" class="Arr (strict)"(error in=w346, "Value"=w337) -> ()  [unwired: 1 in, 2 out]
        n220 = property on="Temp 2" class="Arr (strict)"(error in=w345, "Value"=w336) -> ()  [unwired: 1 in, 2 out]
        n221 = property on="Heater Temp" class="Arr (strict)"(error in=w344, "Value"=w334) -> ()  [unwired: 1 in, 2 out]
        n222 = property on="Time for Temp" class="Arr (strict)"(error in=w352, "Value"=w335) -> ()  [unwired: 1 in, 2 out]
        n223 = Bundle(w335, w337) -> (w343:cluster{dbl[], dbl[]})  [unwired: 1 in]
        n224 = Bundle(w335, w336) -> (w342:cluster{dbl[], dbl[]})  [unwired: 1 in]
        n225 = Bundle(w335, w334) -> (w341:cluster{dbl[], dbl[]})  [unwired: 1 in]
        n226 = Build Array(w343, w342, w341) -> (w339:cluster{dbl[], dbl[]}[])
        n227 = Less Or Equal?(x=w331, y=-5.0) -> (x <= y?=w332:bool)
        n228 = case shown="True" w332 {
          tunnel: w331 -> [_ w367]
          tunnel: [FALSE w365] -> w330
          tunnel: [FALSE w364] -> w329
          frame False {
          }
          frame True {
            n229 = Less Or Equal?(x=w367, y=-20.0) -> (x <= y?=w366:bool)
            n230 = case shown="False" w366 {
              tunnel: [FALSE TRUE] -> w365
              tunnel: [TRUE TRUE] -> w364
              frame False {
              }
              frame True {
              }
            }
          }
        }
        n231 = property on="Interior Temperature" class="XYGraph (strict)"(error in=w340, "Value"=w339) -> (error out=w338:errorcluster)  [unwired: 1 in, 1 out]
        n232 = property on="Low Interior Temperature" class="Bool (strict)"("Value"=w329) -> ()  [unwired: 2 in, 2 out]
        n233 = property on="Critically Low Interior Temperature" class="Bool (strict)"("Value"=w330) -> ()  [unwired: 2 in, 2 out]
      }
      event "Atmospheric Pressure": Value Change {
        n234 = event-data() -> ("NewVal"=w373:dbl)  [unwired: 1 in, 5 out]
        n235 = Get Date/Time In Seconds() -> (seconds since 1Jan1904=w385:timestamp)
        n236 = property on="Start time (minutes)" class="DigNum (strict)"(error in=w387) -> (error out=w380:errorcluster, "Value"=w382:dbl)  [unwired: 1 in, 1 out]
        n237 = To Double Precision Float(number=w385) -> (double precision float=w384:dbl)
        n238 = expression code="x/60"(w384) -> (w383:dbl)
        n239 = Subtract(x=w383, y=w382) -> (x-y=w374:dbl)
        n240 = property on="Atmospheric Pressure" class="XYGraph (strict)"(error in=w380) -> (error out=w377:errorcluster, "Value"=w379:cluster{"X":dbl, "Y":dbl}[])  [unwired: 1 in, 1 out]
        n241 = Bundle By Name(cluster=cluster{"X":dbl, "Y":dbl} {"X"=0.0, "Y"=0.0} ("element"), "X"=w374, "Y"=w373) -> (w378:cluster{"X":dbl, "Y":dbl})
        n242 = Build Array (concatenate)(w379, w378) -> (w376:cluster{"X":dbl, "Y":dbl}[])
        n243 = property on="Atmospheric Pressure" class="XYGraph (strict)"(error in=w377, "Value"=w376) -> (error out=w375:errorcluster)  [unwired: 1 in, 1 out]
      }
      event "Yaw": Value Change {
        n244 = event-data() -> ("NewVal"=w390:dbl)  [unwired: 1 in, 5 out]
        n245 = Get Date/Time In Seconds() -> (seconds since 1Jan1904=w400:timestamp)
        n246 = property on="Start time (minutes)" class="DigNum (strict)"(error in=w404) -> (error out=w396:errorcluster, "Value"=w402:dbl)  [unwired: 1 in, 1 out]
        n247 = To Double Precision Float(number=w400) -> (double precision float=w401:dbl)
        n248 = expression code="x/60"(w401) -> (w399:dbl)
        n249 = Subtract(x=w399, y=w402) -> (x-y=w397:dbl)
        n250 = Bundle By Name(cluster=cluster{"X":dbl, "Y":dbl} {"X"=0.0, "Y"=0.0} ("element"), "X"=w397, "Y"=w390) -> (w393:cluster{"X":dbl, "Y":dbl})
        n251 = property on="Yaw" class="XYGraph (strict)"(error in=w396) -> (error out=w395:errorcluster, "Value"=w392:cluster{"X":dbl, "Y":dbl}[])  [unwired: 1 in, 1 out]
        n252 = Build Array (concatenate)(w392, w393) -> (w391:cluster{"X":dbl, "Y":dbl}[])
        n253 = property on="Yaw" class="XYGraph (strict)"(error in=w395, "Value"=w391) -> (error out=w389:errorcluster)  [unwired: 1 in, 1 out]
      }
      event "Pitch": Value Change {
        # "Get the current time in minutes"
        n254 = event-data() -> ("NewVal"=w406:dbl)  [unwired: 1 in, 5 out]
        n255 = property on="Start time (minutes)" class="DigNum (strict)"(error in=w428) -> (error out=w415:errorcluster, "Value"=w423:dbl)  [unwired: 1 in, 1 out]
        n256 = Get Date/Time In Seconds() -> (seconds since 1Jan1904=w425:timestamp)
        n257 = property on="Roll" class="DigNum (strict)"() -> ("Value"=w405:dbl)  [unwired: 2 in, 2 out]
        n258 = To Double Precision Float(number=w425) -> (double precision float=w426:dbl)
        n259 = expression code="x/60"(w426) -> (w424:dbl)
        n260 = property on="Time for Orientation" class="Arr (strict)"() -> (error out=w422:errorcluster, "Value"=w421:dbl[])  [unwired: 2 in, 1 out]
        n261 = property on="Pitch Array" class="Arr (strict)"() -> (error out=w419:errorcluster, "Value"=w416:dbl[])  [unwired: 2 in, 1 out]
        n262 = property on="Roll Array" class="Arr (strict)"() -> (error out=w418:errorcluster, "Value"=w417:dbl[])  [unwired: 2 in, 1 out]
        n263 = Subtract(x=w424, y=w423) -> (x-y=w420:dbl)
        n264 = Build Array (concatenate)(w416, w406) -> (w412:dbl[])
        n265 = Build Array (concatenate)(w417, w405) -> (w411:dbl[])
        n266 = Build Array (concatenate)(w421, w420) -> (w410:dbl[])
        n267 = property on="Time for Orientation" class="Arr (strict)"(error in=w422, "Value"=w410) -> ()  [unwired: 1 in, 2 out]
        n268 = property on="Pitch Array" class="Arr (strict)"(error in=w419, "Value"=w412) -> ()  [unwired: 1 in, 2 out]
        n269 = property on="Roll Array" class="Arr (strict)"(error in=w418, "Value"=w411) -> ()  [unwired: 1 in, 2 out]
        n270 = Bundle(w410, w412) -> (w409:cluster{dbl[], dbl[]})  [unwired: 1 in]
        n271 = Bundle(w410, w411) -> (w408:cluster{dbl[], dbl[]})  [unwired: 1 in]
        n272 = Build Array(w409, w408) -> (w407:cluster{dbl[], dbl[]}[])
        n273 = property on="Pitch/Roll" class="XYGraph (strict)"(error in=w415, "Value"=w407) -> (error out=w414:errorcluster)  [unwired: 1 in, 1 out]
      }
      event "Relative Humidity": Value Change {
        n274 = event-data() -> ("NewVal"=w430:dbl)  [unwired: 1 in, 5 out]
        n275 = property on="Start time (minutes)" class="DigNum (strict)"(error in=w444) -> (error out=w437:errorcluster, "Value"=w439:dbl)  [unwired: 1 in, 1 out]
        n276 = Get Date/Time In Seconds() -> (seconds since 1Jan1904=w441:timestamp)
        n277 = To Double Precision Float(number=w441) -> (double precision float=w442:dbl)
        n278 = expression code="x/60"(w442) -> (w440:dbl)
        n279 = Subtract(x=w440, y=w439) -> (x-y=w431:dbl)
        n280 = Bundle By Name(cluster=cluster{"X":dbl, "Y":dbl} {"X"=0.0, "Y"=0.0} ("element"), "X"=w431, "Y"=w430) -> (w429:cluster{"X":dbl, "Y":dbl})
        n281 = property on="Relative Humidity" class="XYGraph (strict)"(error in=w437) -> (error out=w436:errorcluster, "Value"=w434:cluster{"X":dbl, "Y":dbl}[])  [unwired: 1 in, 1 out]
        n282 = Build Array (concatenate)(w434, w429) -> (w433:cluster{"X":dbl, "Y":dbl}[])
        n283 = property on="Relative Humidity" class="XYGraph (strict)"(error in=w436, "Value"=w433) -> (error out=w435:errorcluster)  [unwired: 1 in, 1 out]
      }
      event "Save Packets": Value Change {
        n284 = event-data() -> ()  [unwired: 1 in, 6 out]
        n285 = property on="Packet File" class="Path"(error in=w454) -> (error out=w453:errorcluster, "Value"=w451:path)  [unwired: 1 in, 1 out]
        n286 = Empty String/Path?(string/path=w451) -> (empty?=w452:bool)
        n287 = case shown="True" w452 {
          tunnel: w453 -> [w466 w469]
          tunnel: w451 -> [w465 _]
          tunnel: [w457 w469] -> w445
          tunnel: w450 -> [w456 w467]
          tunnel: [w456 w467] -> w449
          tunnel: w448 -> [w455 w468]
          tunnel: [w455 w468] -> w447
          frame False {
            n288 = Open/Create/Replace File(file path (use dialog)=w465, error in=w466, operation (0:open)=T3."replace or create") -> (refnum out=w460:refnum<file>, error out=w463:errorcluster)  [unwired: 3 in, 1 out]
            n289 = property on="Packets Recieved" class="Str"(error in=w463) -> (error out=w462:errorcluster, "Value"=w461:string)  [unwired: 1 in, 1 out]
            n290 = Write to Text File(file (use dialog)=w460, text=w461, error in=w462) -> (refnum out=w458:refnum<file>, error out=w459:errorcluster)  [unwired: 1 in, 1 out]
            n291 = Close File(refnum=w458, error in=w459) -> (error out=w457:errorcluster)  [unwired: 1 out]
          }
          frame True {
          }
        }
        n292 = invoke on="Save Packets" class="Bool" method="Reinit To Default"(error in=w445) -> (error out=w446:errorcluster)  [unwired: 2 in, 2 out]
      }
    }
  }
  n293 = VISA Close(VISA resource name=w39, error in (no error)=w45) -> (error out=w33:errorcluster)
  n294 = Close File(refnum=w32, error in=w33) -> (error out=→"error out":errorcluster)  [unwired: 1 out]
